vi "Start and wait for Configured.vi"(6 "Timeout(1000)":i32=1000, 8 "error in":errorcluster, 10 "DB-Engine":refnum<class "DB-Interface.lvclass">, 11 "Config Section":string) -> (0 "error out":errorcluster, 3 "Module ID":i32)   [LabVIEW 2022 SP3, in "hse-db.lvlib" / "DB_CONNECTOR.lvlib"]
doc: "____\nHAMPEL SOFTWARE ENGINEERING v1.4.0 (2023-12-19 09:52)"
uses:
  DB_CONNECTOR.lvlib
  DB-Interface/DB-Interface.lvclass
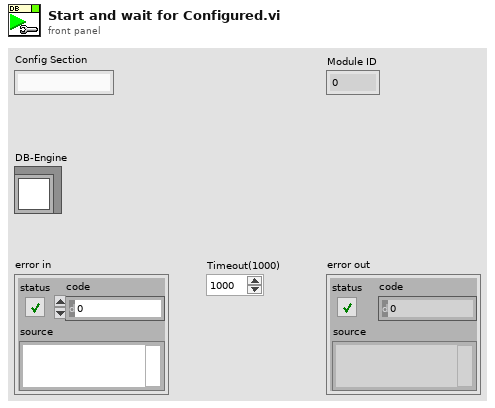
[diagram p1: front panel]
types:
  T1 = typedef "hse-db.lvlib/DB_CONNECTOR.lvlib/Broadcast Events--cluster.ctl" = cluster{"Module Did Init":refnum<user-event>, "Status Updated":refnum<user-event>, "Error Reported":refnum<user-event>, "Module Did Stop":refnum<user-event>, "Update Module Execution Status":refnum<user-event>, "Fast Query Reply":refnum<user-event>, "Configured and Connected":refnum<user-event>}
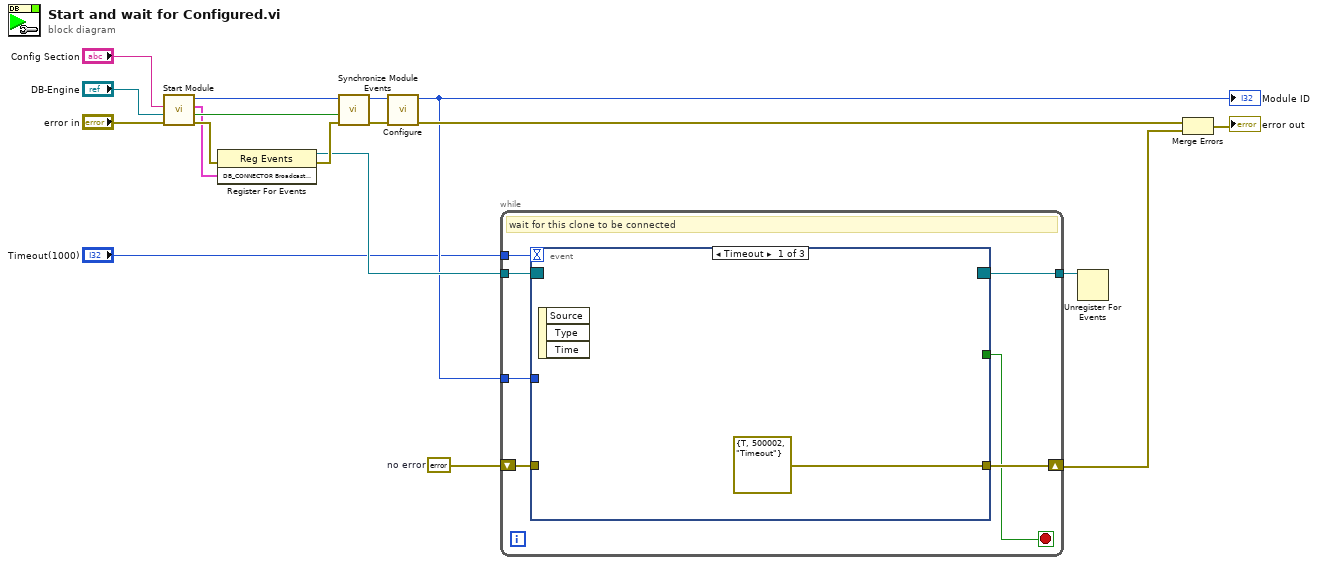
[diagram p0: block diagram]
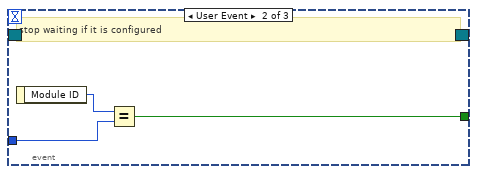
[diagram p2: hidden frame]
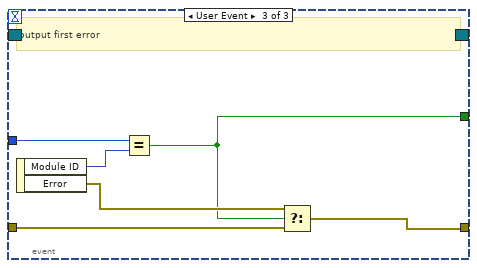
[diagram p3: hidden frame]
diagram:
  w13 = errorcluster {"status"=FALSE, "code"=0, "source"=""}  # no error
  n1 = call "Start Module.vi"("error in (no error)"="error in", "DB-Engine"="DB-Engine", "Config Section"="Config Section") -> ("error out"=w17:errorcluster, "Wait for Event Sync?"=w10:bool, "DB_CONNECTOR Broadcast Events"=w7:T1, "Module ID"=w4:i32)  [unwired: 5 in]
  n2 = register-events(error in=w17, w7) -> (reference out=w5:refnum<event-registration>, error out=w16:errorcluster)  [unwired: 1 in]
  n3 = call "Synchronize Module Events.vi"("error in (no error)"=w16, "Wait for Event Sync?"=w10, "Module ID"=w4) -> ("error out"=w15:errorcluster, "Module ID (dup)"=w6:i32)  [unwired: 7 in]
  n4 = call "Configure.vi"("error in (no error)"=w15, "Module ID"=w6) -> ("error out"=w14:errorcluster, "Module ID (dub)"=w2:i32)  [unwired: 8 in]
  "Module ID" <- w2
  n5 = while {
    tunnel: w5 -> [w23]
    tunnel: w2 -> [w22]
    tunnel: [w20] -> w3
    shift-right: [w24] -> w11
    shift-left: w13 -> [w25]
    tunnel: "Timeout(1000)" -> [w19]
    stop <- w21 stop-if-true
    # "wait for this clone to be connected"
    n6 = event shown="[0] Timeout" {
      selector: w23 -> [_ _ _]
      dyn-events: [_ _ _] -> w20
      timeout: w19 -> [_ _ _]
      tunnel: w22 -> [_ w29 w32]
      tunnel: [_ w27 w30] -> w21
      tunnel: w25 -> [_ _ w34]
      tunnel: [errorcluster {"status"=TRUE, "code"=500002, "source"="Timeout"} ("error") _ w33] -> w24
      event Timeout {
        n7 = event-data() -> ()  [unwired: 1 in, 3 out]
      }
      event User Event {
        # "stop waiting if it is configured"
        n8 = event-data() -> ("Module ID"=w28:i32)  [unwired: 1 in]
        n9 = Equal?(x=w28, y=w29) -> (x = y?=w27:bool)
      }
      event User Event {
        # "output first error"
        n10 = event-data() -> ("Module ID"=w31:i32, "Error"=w35:errorcluster)  [unwired: 1 in]
        n11 = Equal?(x=w32, y=w31) -> (x = y?=w30:bool)
        n12 = Select(t=w35, s=w30, f=w34) -> (s? t:f=w33:errorcluster)
      }
    }
  }
  n13 = Unregister For Events(event registration refnum=w3) -> ()  [unwired: 1 in, 1 out]
  n14 = Merge Errors(w14, w11) -> (→"error out":errorcluster)
